vi "CMD_FINDFID.vi"(6 "Gantry in":refnum<class "Gantry Class.lvclass">, 8 "error in (no error)":errorcluster, 10 "Arguments":string[](array[string]), 11 "gScript Interpreter in":refnum<class "gScript Interpreter.lvclass">) -> (0 "error out":errorcluster, 3 "gScript Interpreter out":refnum<class "gScript Interpreter.lvclass">, 4 "Gantry out":refnum<class "Gantry Class.lvclass">)   [LabVIEW 2017, in "gScript Interpreter.lvclass"]
uses:
  gScript Interpreter.lvclass
  Shared Components/Gantry Class/Gantry Class.lvclass
  Shared Components/CameraTool Class/CameraTool Class.lvclass
  C:/Users/User/Desktop/pixel-gantry-control/Gantry/Shared Components/Gantry Class/Gantry Class.lvclass
  Shared Components/Vec3d Class/Vec3d Class.lvclass
  <vilib>/Utility/error.llb/Error Cluster From Error Code.vi
  <vilib>/ErrorRing/Error Ring.xnode
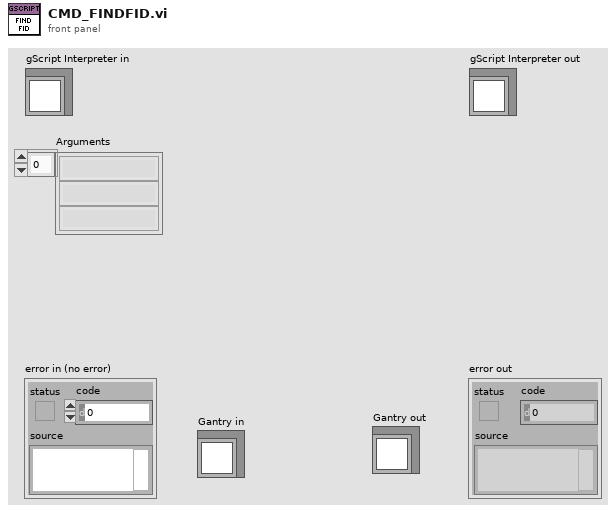
[diagram p1: front panel]
types:
  T1 = typedef "Physical Image.ctl" = cluster{"Image Position":refnum<class "Vec3d Class.lvclass">, "Image Reference":T2, "Field of View":cluster{"x(mm)":dbl, "y(mm)":dbl}}
  T2 = typedef "IMAQ Image.ctl" = refnum<image>
  T3 = typedef "Fiducial with Source.ctl" = cluster{"Fiducial Image Coordinate":refnum<class "Vec3d Class.lvclass">, "Fiducial Source":enum16{"Pattern Recognition", "User", "Error", "Default"}}
  T4 = enum16{"Pattern Recognition", "User", "Error", "Default"}
  T5 = typedef "Memory Cell.ctl" = cluster{"type":T6, "x":dbl, "y":dbl, "z":dbl, "w":dbl}
  T6 = typedef "Memory Cell Type Enum.ctl" = enum16{"integer", "float", "vector", "rotation"}
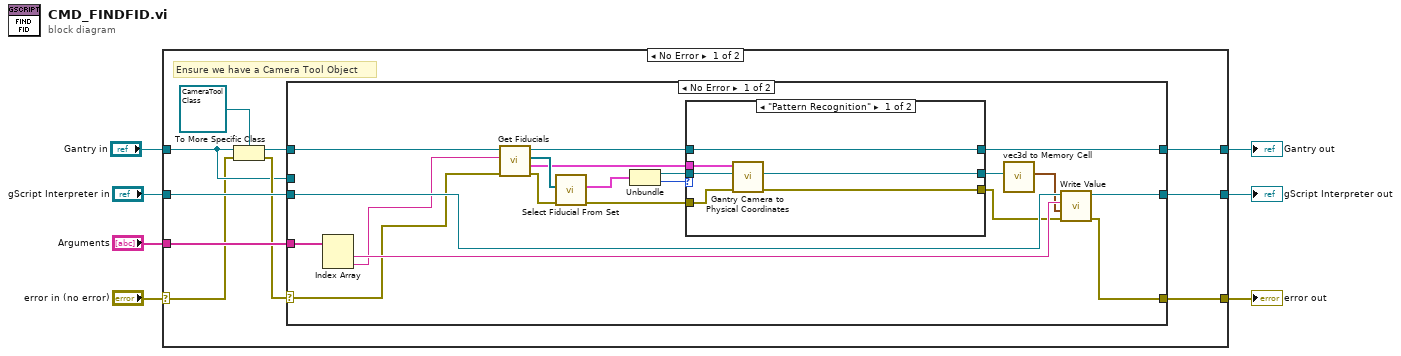
[diagram p0: block diagram]
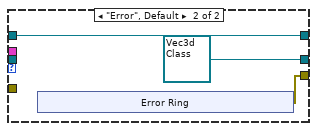
[diagram p2: hidden frame]
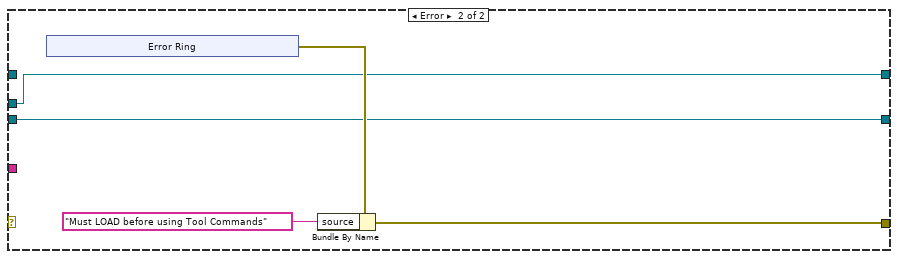
[diagram p3: hidden frame]
diagram:
  n1 = case shown="No Error" "error in (no error)" {
    selector: "error in (no error)" -> [w9 w62]
    tunnel: [w13 w62] -> w6
    tunnel: [w15 w61] -> w4
    tunnel: "gScript Interpreter in" -> [w16 w61]
    tunnel: "Arguments" -> [w17 _]
    tunnel: "Gantry in" -> [w10 w60]
    tunnel: [w14 w60] -> w1
    frame No Error {
      # "Ensure we have a Camera Tool Object"
      n2 = To More Specific Class(target class=refnum<class "CameraTool Class.lvclass"> refnum ("CameraTool Class.lvclass"), reference=w10, error in=w9) -> (specific class reference=w11:refnum<class "CameraTool Class.lvclass">, error out=w12:errorcluster)
      n3 = case shown="No Error" w12 {
        selector: w12 -> [w19 _]
        tunnel: w17 -> [w37 _]
        tunnel: w16 -> [w26 w52]
        tunnel: [w21 w52] -> w15
        tunnel: [w27 w51] -> w14
        tunnel: [w20 w53] -> w13
        tunnel: w11 -> [w36 _]
        tunnel: w10 -> [_ w51]
        frame No Error {
          n4 = Index Array(array=w37) -> (element #1=w25:string, element #2=w18:string)  [unwired: 2 in]
          n5 = call "Get Fiducials.vi"("error in"=w19, "Fiducial Type"=w18, "CameraTool In"=w36) -> ("error out"=w34:errorcluster, "Fiducial Image"=w29:T1, "Fiducial Image Positions"=w35:refnum<class "Vec3d Class.lvclass">[], "CameraTool Out"=w28:refnum<class "CameraTool Class.lvclass">)  [unwired: 3 in]
          n6 = call "Select Fiducial From Set.vi"("error in"=w34, "Fiducial Centers"=w35) -> ("error out"=w30:errorcluster, "Fiducial with Source"=w33:T3)  [unwired: 8 in]
          n7 = Unbundle(w33) -> ("Fiducial Image Coordinate"=w31:refnum<class "Vec3d Class.lvclass">, "Fiducial Source"=w32:T4)
          n8 = case shown="\"Pattern Recognition\"" w32 {
            tunnel: w31 -> [w42 _]
            tunnel: w30 -> [w41 _]
            tunnel: w29 -> [w43 _]
            tunnel: w28 -> [w40 w46]
            tunnel: [w40 w46] -> w27
            tunnel: [w39 refnum<class "Vec3d Class.lvclass"> refnum ("Global Coordinate")] -> w23
            tunnel: [w38 w45] -> w24
            frame "Pattern Recognition" {
              n9 = call "Gantry Camera to Physical Coordinates.vi"("error in"=w41, "Image Coordinate"=w42, "Physical Image"=w43) -> ("error out"=w38:errorcluster, "Global Coordinate"=w39:refnum<class "Vec3d Class.lvclass">)  [unwired: 6 in, 1 out]
            }
            frame "Error", Default {
              n10 = xnode "Error Ring"() -> ("error out"=w45:errorcluster)
            }
          }
          n11 = call "vec3d to Memory Cell.vi"("Vec3d in"=w23) -> ("Memory Cell"=w22:T5)  [unwired: 10 in]
          n12 = call-dynamic "Write Value.vi"("error in (no error)"=w24, "Value"=w22, "Address"=w25, "gScript Interpreter in"=w26) -> ("error out"=w20:errorcluster, "gScript Interpreter out"=w21:refnum<class "gScript Interpreter.lvclass">)  [unwired: 6 in]
        }
        frame Error {
          n13 = xnode "Error Ring"() -> ("error out"=w55:errorcluster)
          n14 = Bundle By Name(cluster=w55, "source"="Must LOAD before using Tool Commands") -> (w53:errorcluster)
        }
      }
    }
    frame Error {
    }
  }
  "error out" <- w6
  "gScript Interpreter out" <- w4
  "Gantry out" <- w1
